vi "Ex_Read.vi"() -> ()   [LabVIEW 2015]
doc: "X-CAN example VI that continually reads data from the X-CAN device using an X-CAN Session. If no data is on the X-CAN device, the VI will clear the error, set Data Ready? flag to false and not update the X-CAN LEDs."
uses:
  <vilib>/Stratom, Inc/X-CAN for myRIO (API)/X-CAN Class/Type Definitions/CANFrame.ctl
  <vilib>/Stratom, Inc/X-Modules for myRIO/Type Defs/MXPChannel.ctl
  <vilib>/Stratom, Inc/X-CAN for myRIO (API)/X-CAN Class/Type Definitions/CAN_Speed.ctl
  <vilib>/Platform/TimedLoop/XDataNode/timing_clust.ctl
  <vilib>/Platform/TimedLoop/XDataNode/nitl_modes.ctl
  <vilib>/Platform/TimedLoop/XDataNode/wakeup.ctl
  <vilib>/Platform/TimedLoop/XDataNode/XDataNode.xnode
  <vilib>/Stratom, Inc/X-CAN for myRIO (API)/X-CAN Class/X-CAN.lvclass
  <vilib>/Platform/TimedLoop/XDataNode/XDNodeRunTimeDep.lvlib
panel:
  out "Data Ready?":bool
  out "CAN Frame":T1 {"payload" format="%x"; "timestamp" format="%<%I:%M:%S%8u %p\n%x>T"; "identifier" format="%x"}
  in  "Stop Button":bool
  # "X-CAN Read"
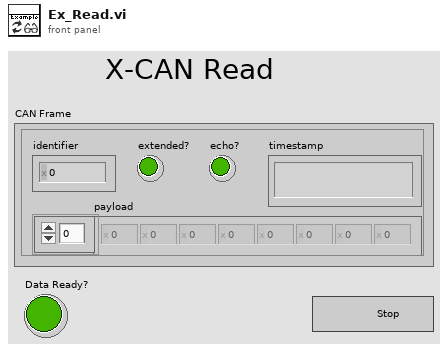
[diagram p1: front panel]
types:
  T1 = typedef "X-CAN.lvclass/CANFrame.ctl" = cluster{"identifier":u32, "extended?":bool, "echo?":bool, "payload":u8[], "timestamp":timestamp}
  T2 = typedef "X-CAN.lvclass/CAN_Speed.ctl" = u8
  T3 = typedef "MXPChannel.ctl" = enum16{"A/MXP", "B/MXP"}
  T4 = typedef "XDNodeRunTimeDep.lvlib/timing_clust.ctl" = cluster{"Expected End [f-1]":u64, "Actual End [f-1]":u64, "Finished Late? [f-1]":bool, "Expected End [i-1]":u64, "Actual End [i-1]":u64, "Finished Late? [i-1]":bool, "Expected Start [i]":u64, "Actual Start [i]":u64, "Expected Start [f]":u64, "Actual Start [f]":u64, "Source Name":string, "Structure Name":string, "Period":i64, "Deadline":i64, "Offset":i64, "Start":i64, "Priority":i32, "Timeout":i32, "Mode":T5, "Wakeup Reason":T6, "Error":errorcluster, "Source Type":string, "Secondary Source Type":string, "Global End Time":u64, "Global Start Time":u64, "Frame Duration":u64, "Iteration Duration":u64, "Assigned CPU":i32, "I/O Scan Engine Mode":u32}
  T5 = typedef "XDNodeRunTimeDep.lvlib/nitl_modes.ctl" = enum32{"No Change", "Process missed periods, maintain original phase", "Discard missed periods, maintain original phase", "Process missed periods, ignore original phase", "Discard missed periods, ignore original phase"}
  T6 = typedef "XDNodeRunTimeDep.lvlib/wakeup.ctl" = enum32{"Normal", "Aborted", "Asynchronous wakeup", "Timing source error", "Timed loop error", "Timeout"}
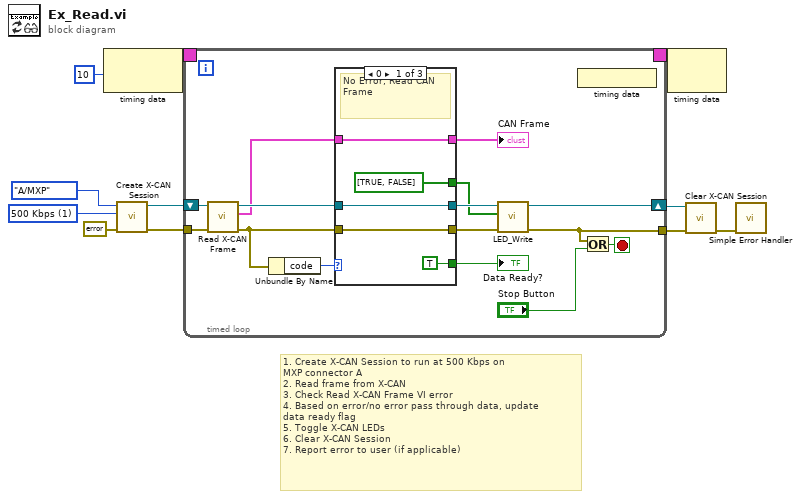
[diagram p0: block diagram]
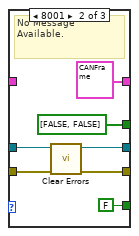
[diagram p2: hidden frame]
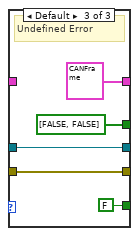
[diagram p3: hidden frame]
diagram:
  w6 = T2 1 items=["125 Kbps"=7, "250 Kbps"=3, "500 Kbps"=1, "1000 Kbps"=0, "95.238 Kbps"=6] ("CAN Speed [Kbps]")
  # "1. Create X-CAN Session to run at 500 Kbps on \nMXP connector A\n2. Read frame from X-CAN\n3. Check Read X-CAN Frame VI error\n4. Based on error/no error pass through data, update\ndata ready flag \n5. Toggle X-CAN LEDs \n6. Clear X-CAN Session\n7. Report error to user (if applicable)"
  n1 = node-c288(i64 10 ("Period")) -> (w11:T4)
  n2 = call <vilib>:"Create X-CAN Session.vi"("error in (no error)"=errorcluster {"status"=FALSE, "code"=0, "source"=""}, "CAN Speed [Kbps]"=w6, "MXP Channel"=MXPChannel."A/MXP") -> ("error out"=w9:errorcluster, "X-CAN Session out"=w2:refnum<class "X-CAN.lvclass">)  [unwired: 7 in]
  n3 = timed-loop {
    timing: w11 -> [_]
    timing-out: [_] -> w10
    tunnel: w9 -> [w13]
    shift-right: [w23] -> w4
    shift-left: w2 -> [w14]
    tunnel: [w22] -> w5
    stop <- w25 stop-if-true
    n4 = call <vilib>:"Read X-CAN Frame.vi"("error in"=w13, "X-CAN Session in"=w14) -> ("error out"=w20:errorcluster, "CAN Frame"=w16:T1, "X-CAN Session out"=w19:refnum<class "X-CAN.lvclass">)  [unwired: 7 in]
    n5 = Unbundle By Name(w20) -> ("code"=w21:i32)
    n6 = case shown="0" w21 {
      tunnel: w20 -> [w31 w36 w41]
      tunnel: w19 -> [w30 w34 w42]
      tunnel: [w30 w34 w42] -> w26
      tunnel: [w31 w35 w41] -> w18
      tunnel: [TRUE FALSE FALSE] -> w17
      tunnel: w16 -> [w28 _ _]
      tunnel: [w28 T1 {"identifier"=0, "extended?"=FALSE, "echo?"=FALSE, "payload"=[], "timestamp"=timestamp(0 s since 1904-01-01)} ("CAN Frame") T1 {"identifier"=0, "extended?"=FALSE, "echo?"=FALSE, "payload"=[], "timestamp"=timestamp(0 s since 1904-01-01)} ("CAN Frame")] -> w15
      tunnel: [bool[] [TRUE, FALSE] ("LED Values") bool[] [FALSE, FALSE] ("LED Values") bool[] [FALSE, FALSE] ("LED Values")] -> w12
      frame 0 {
        # "No Error, Read CAN Frame"
      }
      frame 8001 {
        # "No Message Available."
        n7 = call <vilib>:"Clear Errors.vi"("error in (no error)"=w36) -> ("error out"=w35:errorcluster)  [unwired: 5 in, 1 out]
      }
      frame Default {
        # "Undefined Error"
      }
    }
    "Data Ready?" <- w17
    "CAN Frame" <- w15
    n8 = call <vilib>:"LED_Write.vi"("error in"=w18, "LED Values"=w12, "X-CAN in"=w26) -> ("error out"=w22:errorcluster, "X-CAN out"=w23:refnum<class "X-CAN.lvclass">)  [unwired: 7 in]
    n9 = node-c288() -> ()  [unwired: 1 out]
    n10 = Or(x=w22, y="Stop Button") -> (x .or. y?=w25:bool)
  }
  n11 = node-c288(w10) -> ()  [unwired: 1 out]
  n12 = call <vilib>:"Clear X-CAN Session.vi"("error in (no error)"=w5, "X-CAN Session in"=w4) -> ("error out"=w3:errorcluster)  [unwired: 9 in]
  n13 = call <vilib>:"Simple Error Handler.vi"("error in (no error)"=w3) -> ()  [unwired: 4 in, 5 out]
